vi "Read Pixel.vi"(8 "error in (no error)":errorcluster, 10 "indices":T1, 11 "Picture in":refnum<class "Picture.lvclass">) -> (0 "error out":errorcluster, 2 "Color":u32, 3 "Picture out":refnum<class "Picture.lvclass">)   [LabVIEW 2018, in "Picture.lvclass"]
uses:
  Picture.lvclass
  Coords.ctl
  Picture.lvclass/Picture.ctl
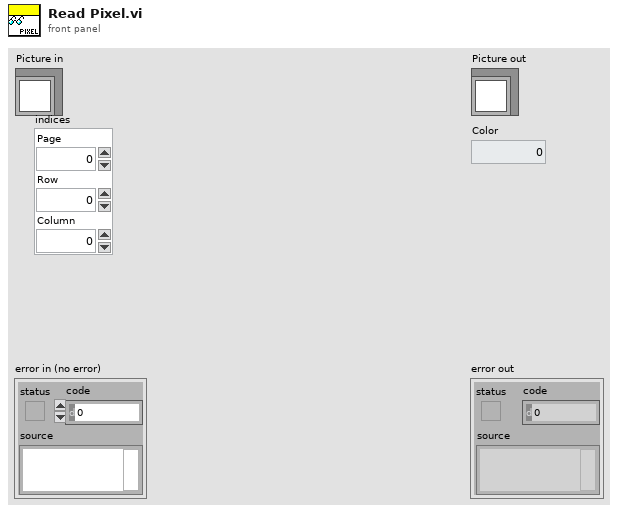
[diagram p1: front panel]
types:
  T1 = typedef "Coords.ctl" = cluster{"Page":i32, "Row":i32, "Column":i32}
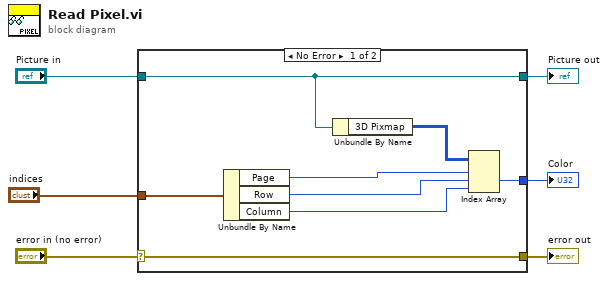
[diagram p0: block diagram]
diagram:
  n1 = case shown="No Error" "error in (no error)" {
    selector: "error in (no error)" -> [w7 w15]
    tunnel: [w7 w15] -> w5
    tunnel: [w8 w16] -> w3
    tunnel: "Picture in" -> [w8 w16]
    tunnel: [w14 _] -> w2
    tunnel: "indices" -> [w12 _]
    frame No Error {
      n2 = Unbundle By Name(w12) -> ("Page"=w9:i32, "Row"=w11:i32, "Column"=w10:i32)
      n3 = Unbundle By Name(w8) -> ("3D Pixmap"=w13:u32[][][])
      n4 = Index Array(array=w13, index (dim 0)=w9, index (dim 1)=w11, index (dim 2)=w10) -> (element=w14:u32)
    }
    frame Error {
    }
  }
  "error out" <- w5
  "Picture out" <- w3
  "Color" <- w2
